vi "Test Properties Report.vi"() -> ()   [LabVIEW 2013]
uses:
  classes/Test Result/Node Results (Extended).ctl
  classes/Test Result/Test Node (Extended).ctl
  classes/Test Result/Test Registration Data.ctl
  classes/Test Result/Assert Event Data (Extended).ctl
  classes/Test Suite/Test Suite.lvclass
  classes/Test Result/Test Result.lvclass
panel:
  out "Test Results":T1[](array[typedef])
  in  "error in (no error)":errorcluster
  out "error out":errorcluster
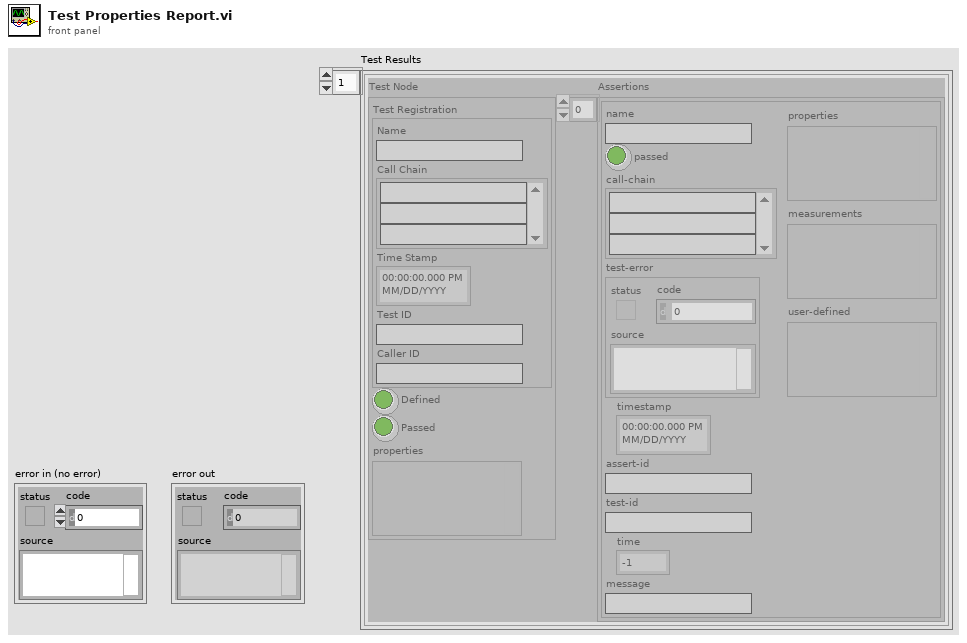
[diagram p1: front panel]
types:
  T1 = typedef "Caraya.lvlib/Test Result.lvclass/Node Results (Extended).ctl" = cluster{"Test Node":T2, "Assertions":T4[]}
  T2 = typedef "Caraya.lvlib/Test Result.lvclass/Test Node (Extended).ctl" = cluster{"Test Registration":T3, "Defined":bool, "Passed":bool, "properties":variant}
  T3 = typedef "Caraya.lvlib/Test Result.lvclass/Test Registration Data.ctl" = cluster{"Name":string, "Call Chain":string[], "Time Stamp":timestamp, "Test ID":string, "Caller ID":string}
  T4 = typedef "Caraya.lvlib/Test Result.lvclass/Assert Event Data (Extended).ctl" = cluster{"name":string, "passed":bool, "call-chain":string[], "test-error":errorcluster, "timestamp":timestamp, "assert-id":string, "test-id":string, "time":dbl, "message":string, "properties":variant, "measurements":variant, "user-defined":variant}
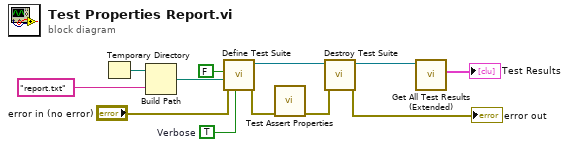
[diagram p0: block diagram]
diagram:
  w9 = TRUE  # Verbose
  n1 = Temporary Directory() -> (w11:path)
  n2 = Build Path(base path=w11, name or relative path="report.txt") -> (appended path=w10:path)
  n3 = call "Define Test Suite.vi"("Verbose (F)"=w9, "error in (no error)"="error in (no error)", "Report Path"=w10, "Interactive"=FALSE) -> ("error out"=w2:errorcluster, "Test Suite"=w8:refnum<class "Test Suite.lvclass">)  [unwired: 5 in, 1 out]
  n4 = call "Test Assert Properties.vi"("error in (no error)"=w2) -> ("error out"=w4:errorcluster)  [unwired: 10 in]
  n5 = call-dynamic "Destroy Test Suite.vi"("error in (no error)"=w4, "Test Suite in"=w8) -> ("error out"=→"error out":errorcluster, "Test Suite Results"=w7:refnum<class "Test Result.lvclass">)  [unwired: 8 in]
  n6 = call "Get All Test Results (Extended).vi"("Test Result in"=w7) -> ("Test Results"=→"Test Results":T1[])  [unwired: 8 in, 2 out]
